vi "Convert DAC to Mass.vi"(1 "Calibration Table":dbl[][](array[numeric]) format="%.2f", 2 "DAC":dbl format="%.2f") -> (0 "Mass":dbl format="%.2f")   [LabVIEW 2018]
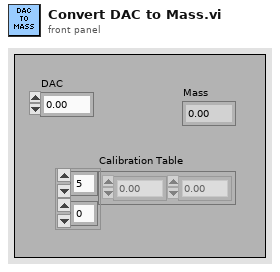
[diagram p1: front panel]
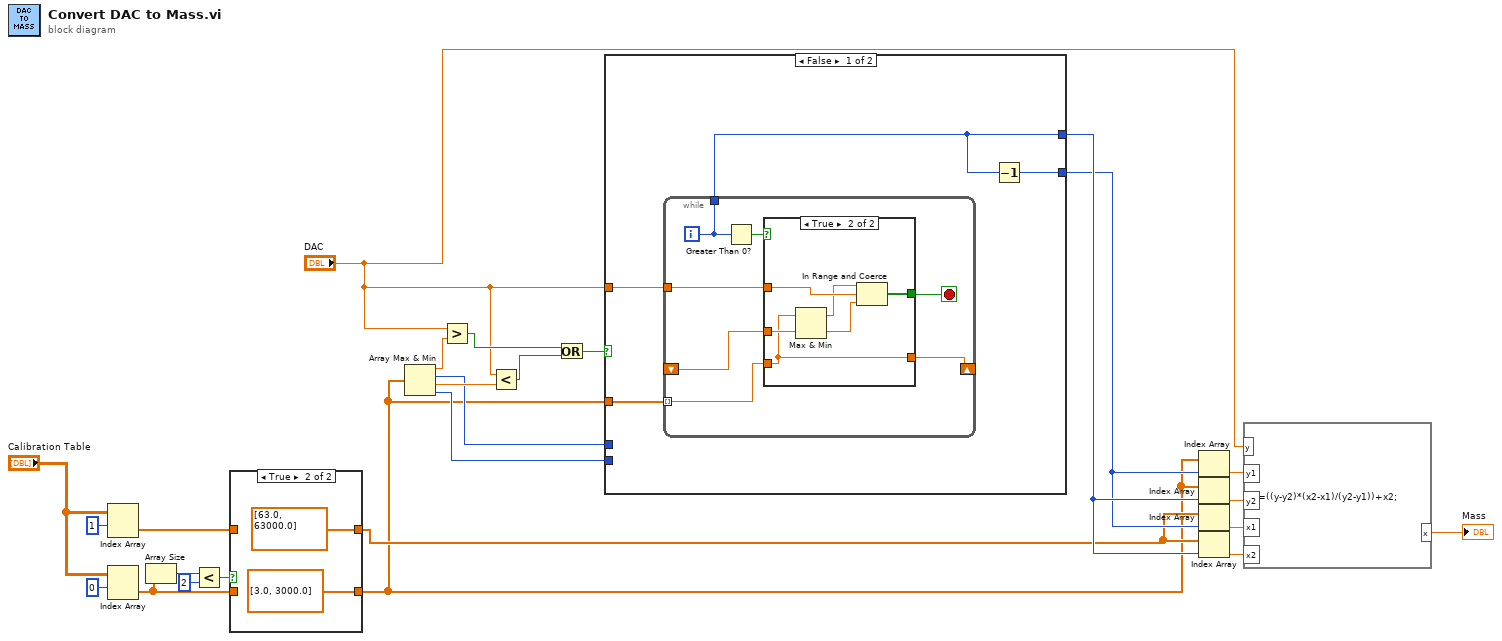
[diagram p0: block diagram]
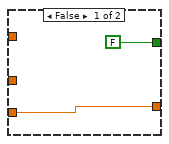
[diagram p2: hidden frame]
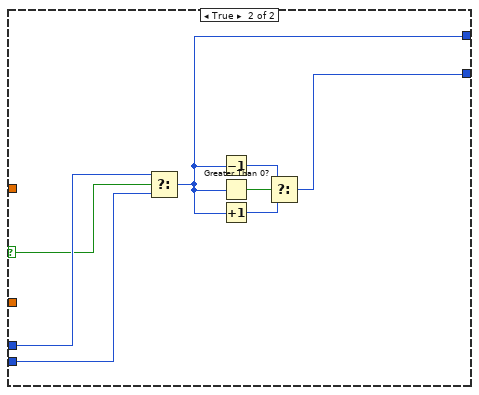
[diagram p3: hidden frame]
diagram:
  n1 = Index Array(array="Calibration Table", index (row)=1) -> (element=w21:dbl[])  [unwired: 1 in]
  n2 = Index Array(array="Calibration Table", index (row)=0) -> (element=w22:dbl[])  [unwired: 1 in]
  n3 = Array Size(array=w22) -> (size(s)=w25:i32)
  n4 = Less?(x=w25, y=2) -> (x < y?=w23:bool)
  n5 = case shown="True" w23 {
    tunnel: w22 -> [w26 _]
    tunnel: w21 -> [w27 _]
    tunnel: [w26 dbl[] [3.0, 3000.0]] -> w6
    tunnel: [w27 dbl[] [63.0, 63000.0]] -> w7
    frame False {
    }
    frame True {
    }
  }
  n6 = Array Max & Min(array=w6) -> (max value=w17:dbl, max index (indices)=w12:i32, min value=w14:dbl, min index (indices)=w11:i32)
  n7 = Greater?(x="DAC", y=w17) -> (0:w15:bool)
  n8 = Less?(x="DAC", y=w14) -> (x < y?=w16:bool)
  n9 = Or(x=w15, y=w16) -> (x .or. y?=w13:bool)
  n10 = case shown="False" w13 {
    selector: w13 -> [_ w51]
    tunnel: "DAC" -> [w33 _]
    tunnel: w6 -> [w32 _]
    tunnel: w12 -> [_ w53]
    tunnel: w11 -> [_ w52]
    tunnel: [w31 w50] -> w9
    tunnel: [w30 w49] -> w8
    frame False {
      n11 = while {
        tunnel: w32 -> [w40] mode=indexing
        tunnel: w33 -> [w36]
        shift-right: [w38] -> _
        shift-left: _ -> [w37]
        tunnel: [w34] -> w31
        i -> [w34]
        stop <- w35 stop-if-true
        n12 = Greater Than 0?(x=w34) -> (x > 0?=w39:bool)
        n13 = case shown="True" w39 {
          tunnel: w40 -> [w42 w47]
          tunnel: [w42 w47] -> w38
          tunnel: w37 -> [_ w48]
          tunnel: w36 -> [_ w46]
          tunnel: [FALSE w43] -> w35
          frame False {
          }
          frame True {
            n14 = Max & Min(x=w47, y=w48) -> (max(x,y)=w45:dbl, min(x,y)=w44:dbl)
            n15 = In Range and Coerce(upper limit=w45, x=w46, lower limit=w44) -> (In Range?=w43:bool)  [unwired: 1 out]
          }
        }
      }
      n16 = Decrement(x=w31) -> (x-1=w30:i32)
    }
    frame True {
      n17 = Select(t=w53, s=w51, f=w52) -> (s? t:f=w50:i32)
      n18 = Decrement(x=w50) -> (x-1=w55:i32)
      n19 = Greater Than 0?(x=w50) -> (x > 0?=w56:bool)
      n20 = Increment(x=w50) -> (x+1=w54:i32)
      n21 = Select(t=w55, s=w56, f=w54) -> (s? t:f=w49:i32)
    }
  }
  n22 = Index Array(array=w6, index=w8) -> (element=w5:dbl)
  n23 = Index Array(array=w6, index=w9) -> (element=w4:dbl)
  n24 = Index Array(array=w7, index=w8) -> (element=w3:dbl)
  n25 = Index Array(array=w7, index=w9) -> (element=w2:dbl)
  n26 = formula code="x=((y-y2)*(x2-x1)/(y2-y1))+x2;"("y1"=w5, "y2"=w4, "x1"=w3, "x2"=w2, "y"="DAC") -> ("x"=→"Mass":dbl)
